vi "Process Log Request.vi"(10 "Log Packet":T1, 11 "SessionHandler in":refnum<class "SessionHandler.lvclass">) -> (0 "error out":errorcluster, 3 "SessionHandler out":refnum<class "SessionHandler.lvclass">)   [LabVIEW 2019, in "Network Sink.lvlib" / "SessionHandler.lvclass"]
uses:
  <vilib>/gpm_packages/@cs/event-logger/Source/Network Sink/SessionHandler/SessionHandler.lvclass
  <vilib>/gpm_packages/@cs/event-logger/Source/Composed Log/Types/Log Packet.ctl
  <vilib>/gpm_packages/@cs/event-logger/Source/Composed Log/Types/Log Level.ctl
  <vilib>/gpm_packages/@cs/event-logger/Source/Network Sink/SessionHandler/SessionHandler.lvclass/SessionHandler.ctl
  <vilib>/gpm_packages/@cs/Network-Sink/Source/Network Interface/IMessagingProtocol/IMessagingProtocol.lvclass
  <vilib>/gpm_packages/@cs/event-logger/Source/Composed Log/Composed Log.lvlib
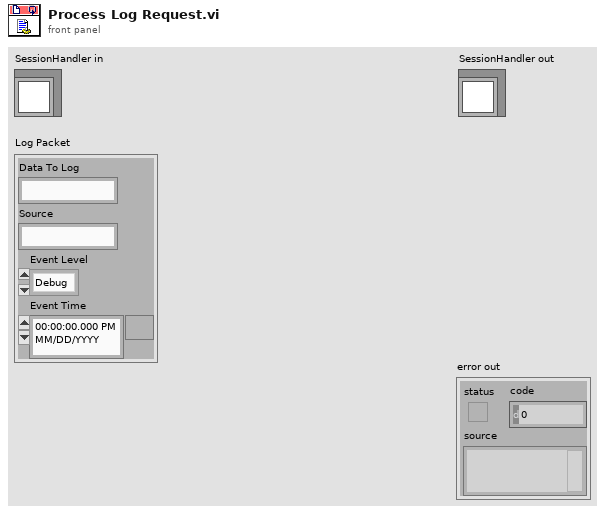
[diagram p1: front panel]
types:
  T1 = typedef "Composed Log.lvlib/Log Packet.ctl" = cluster{"Data To Log":string, "Source":string, "Event Level":T2, "Event Time":timestamp}
  T2 = typedef "Composed Log.lvlib/Log Level.ctl" = enum16{"Debug", "Info", "Warning", "Error", "Critical"}
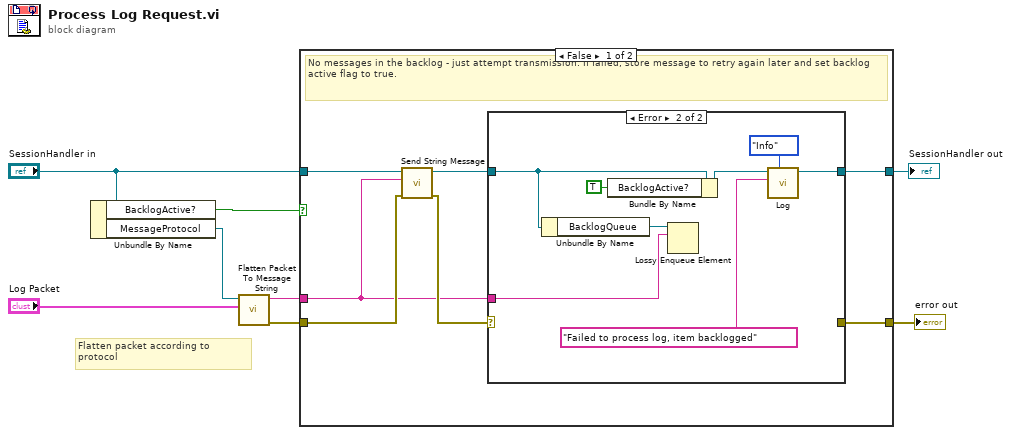
[diagram p0: block diagram]
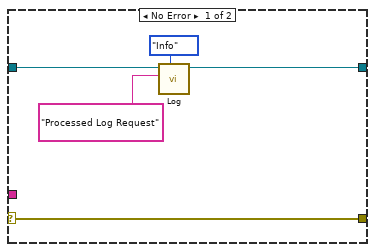
[diagram p2: hidden frame]
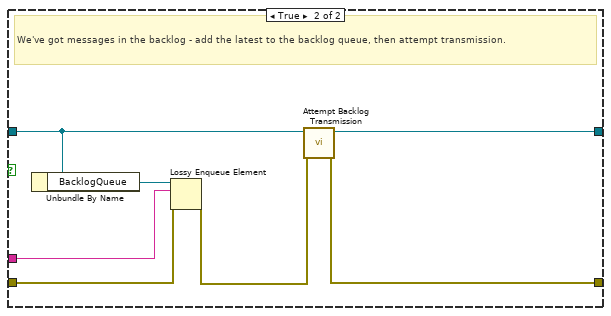
[diagram p3: hidden frame]
diagram:
  # "Flatten packet according to protocol"
  n1 = Unbundle By Name("SessionHandler in") -> ("BacklogActive?"=w2:bool, "MessageProtocol"=w8:refnum<class "IMessagingProtocol.lvclass">)
  n2 = call-dynamic "Flatten Packet To Message String.vi"("Message Packet"="Log Packet", "IMessagingProtocol in"=w8) -> ("error out"=w5:errorcluster, "Packet as Message String"=w3:string)  [unwired: 8 in]
  n3 = case shown="False" w2 {
    tunnel: "SessionHandler in" -> [w15 w33]
    tunnel: w5 -> [w14 w32]
    tunnel: [w11 w29] -> w4
    tunnel: w3 -> [w10 w34]
    tunnel: [w9 w30] -> w1
    frame False {
      # "No messages in the backlog - just attempt transmission. If failed, store message to retry again later and set backlog active flag to true."
      n4 = call <vilib>:"Send String Message.vi"("error in (no error)"=w14, "Data To Write"=w10, "SessionHandler in"=w15) -> ("error out"=w13:errorcluster, "SessionHandler out"=w12:refnum<class "SessionHandler.lvclass">)  [unwired: 7 in]
      n5 = case shown="Error" w13 {
        selector: w13 -> [w20 _]
        tunnel: w12 -> [w19 w28]
        tunnel: [w18 w23] -> w9
        tunnel: [w20 _] -> w11
        tunnel: w10 -> [_ w26]
        frame No Error {
          n6 = call <vilib>:"Log.vi"("Event Level"=Log_Level."Info", "Data To Log"="Processed Log Request", "SessionHandler in"=w19) -> ("SessionHandler out"=w18:refnum<class "SessionHandler.lvclass">)  [unwired: 7 in, 1 out]
        }
        frame Error {
          n7 = Unbundle By Name(w28) -> ("BacklogQueue"=w27:refnum<queue>)
          n8 = Bundle By Name(cluster=w28, "BacklogActive?"=TRUE) -> (w24:refnum<class "SessionHandler.lvclass">)
          n9 = Lossy Enqueue Element(queue=w27, element=w26) -> ()  [unwired: 1 in, 4 out]
          n10 = call <vilib>:"Log.vi"("Event Level"=Log_Level."Info", "Data To Log"="Failed to process log, item backlogged", "SessionHandler in"=w24) -> ("SessionHandler out"=w23:refnum<class "SessionHandler.lvclass">)  [unwired: 7 in, 1 out]
        }
      }
    }
    frame True {
      # "We've got messages in the backlog - add the latest to the backlog queue, then attempt transmission."
      n11 = Unbundle By Name(w33) -> ("BacklogQueue"=w35:refnum<queue>)
      n12 = Lossy Enqueue Element(queue=w35, element=w34, error in (no error)=w32) -> (error out=w31:errorcluster)  [unwired: 3 out]
      n13 = call <vilib>:"Attempt Backlog Transmission.vi"("error in (no error)"=w31, "SessionHandler in"=w33) -> ("error out"=w29:errorcluster, "SessionHandler out"=w30:refnum<class "SessionHandler.lvclass">)  [unwired: 8 in]
    }
  }
  "error out" <- w4
  "SessionHandler out" <- w1
